vi "Write_Read.vi"(8 "error in (no error)":errorcluster, 10 "write visa cmd buffer":string, 11 "PowerSupply_IT6333A in":refnum<class "PowerSupply_IT6333A.lvclass">) -> (0 "error out":errorcluster, 2 "read buffer":string, 3 "PowerSupply_IT6333A out":refnum<class "PowerSupply_IT6333A.lvclass">)   [LabVIEW 2013, in "PowerSupply_IT6333A.lvclass"]
uses:
  PowerSupply_IT6333A.lvclass
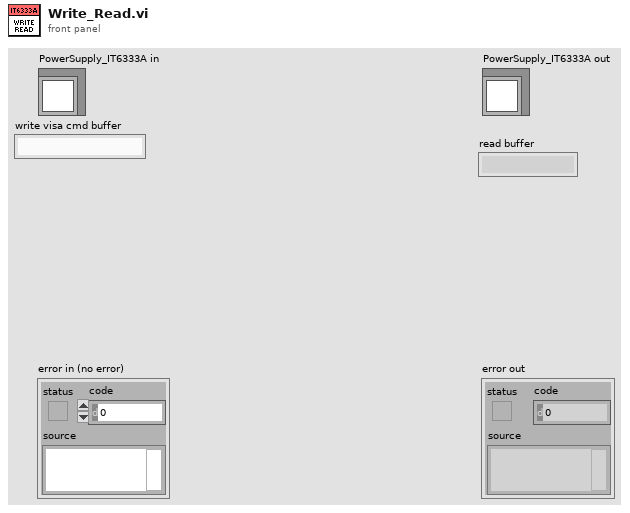
[diagram p1: front panel]
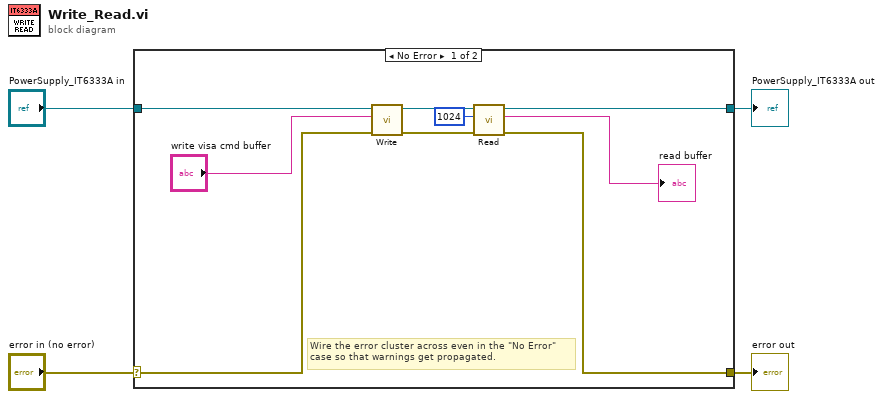
[diagram p0: block diagram]
diagram:
  n1 = case shown="No Error" "error in (no error)" {
    selector: "error in (no error)" -> [w10 w15]
    tunnel: [w9 w15] -> w3
    tunnel: [w12 w14] -> w1
    tunnel: "PowerSupply_IT6333A in" -> [w6 w14]
    frame No Error {
      # "Wire the error cluster across even in the \"No Error\"\ncase so that warnings get propagated."
      n2 = call-dynamic "Write.vi"("error in (no error)"=w10, "write visa cmd buffer"="write visa cmd buffer", "PowerSupply_IT6333A in"=w6) -> ("error out"=w11:errorcluster, "PowerSupply_IT6333A out"=w13:refnum<class "PowerSupply_IT6333A.lvclass">)  [unwired: 7 in]
      n3 = call-dynamic "Read.vi"("error in (no error)"=w11, "byte count"=u32 1024, "PowerSupply_IT6333A in"=w13) -> ("error out"=w9:errorcluster, "read buffer"=→"read buffer":string, "PowerSupply_IT6333A out"=w12:refnum<class "PowerSupply_IT6333A.lvclass">)  [unwired: 6 in]
    }
    frame Error {
    }
  }
  "error out" <- w3
  "PowerSupply_IT6333A out" <- w1
